vi "authorize.vi"() -> (3 "Flickr Ref out":refnum<k24>)   [LabVIEW 2010]
uses:
  C:/Users/telsey/Desktop/Personal Projects/Photobooth/Flickr API/FlickrNet-3.5.0/FlickrNet.dll
  FlickrNet.dll
  <userlib>/_OpenG.lib/md5/md5.llb/MD5 Message Digest (Hexadecimal String)__ogtk.vi
panel:
  out "LastResponse 2":string
  out "LastResponse":string
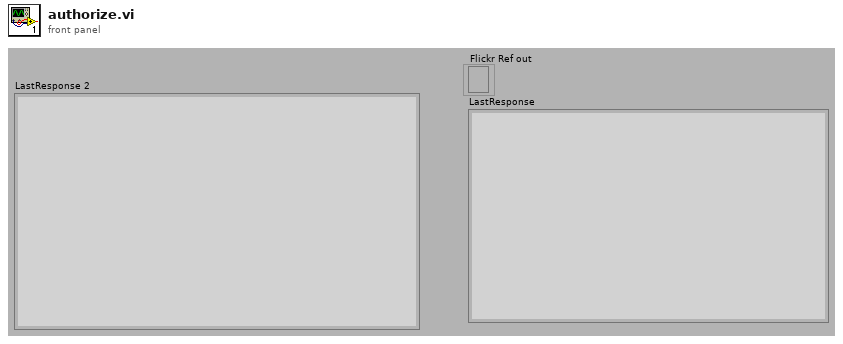
[diagram p1: front panel]
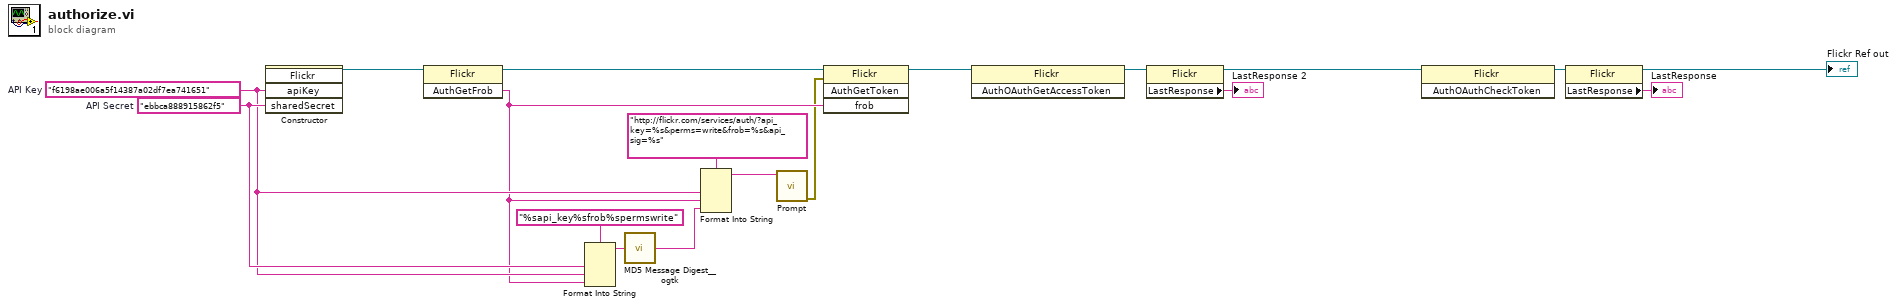
[diagram p0: block diagram]
diagram:
  w17 = "ebbca888915862f5"  # API Secret
  w16 = "f6198ae006a5f14387a02df7ea741651"  # API Key
  n1 = constructor class="Flickr"("apiKey"=w16, "sharedSecret"=w17) -> (reference out=w18:refnum<k24>)  [unwired: 3 in, 4 out]
  n2 = invoke class="Flickr" method="AuthGetFrob"(reference=w18) -> (reference out=w5:refnum<k24>, "AuthGetFrob"=w6:string)  [unwired: 2 in, 1 out]
  n3 = Format Into String(format string="%sapi_key%sfrob%spermswrite", w17, w16, w6) -> (resulting string=w8:string)  [unwired: 2 in, 1 out]
  n4 = call-poly <userlib>:"MD5 Message Digest__ogtk.vi"("Message"=w8) -> ("MD5 Message Digest"=w7:string)
  n5 = Format Into String(format string="http://flickr.com/services/auth/?api_key=%s&perms=write&frob=%s&api_sig=%s", w16, w6, w7) -> (resulting string=w4:string)  [unwired: 2 in, 1 out]
  n6 = call "Prompt.vi"("URL"=w4) -> ("error out"=w3:errorcluster)  [unwired: 10 in]
  n7 = invoke class="Flickr" method="AuthGetToken"(reference=w5, error in=w3, "frob"=w6) -> (reference out=w12:refnum<k24>)  [unwired: 1 in, 3 out]
  n8 = invoke class="Flickr" method="AuthOAuthGetAccessToken"(reference=w12) -> (reference out=w13:refnum<k24>)  [unwired: 2 in, 2 out]
  n9 = property class="Flickr"(reference=w13) -> (reference out=w2:refnum<k24>, "LastResponse"=→"LastResponse 2":string)  [unwired: 1 in, 1 out]
  n10 = invoke class="Flickr" method="AuthOAuthCheckToken"(reference=w2) -> (reference out=w11:refnum<k24>)  [unwired: 2 in, 2 out]
  n11 = property class="Flickr"(reference=w11) -> (reference out=→"Flickr Ref out":refnum<k24>, "LastResponse"=→"LastResponse":string)  [unwired: 1 in, 1 out]
